vi "Clean exp.vi"(8 "error in (no error)":errorcluster, 11 "Control-Client in":refnum<class "Control-Client.lvclass">) -> (0 "error out":errorcluster, 3 "Control-Client out":refnum<class "Control-Client.lvclass">)   [LabVIEW 2019, in "Control-Client.lvclass"]
uses:
  Control-Client.lvclass
  Control-Client.lvclass/Control-Client.ctl
  Experiments/Experiment.lvclass
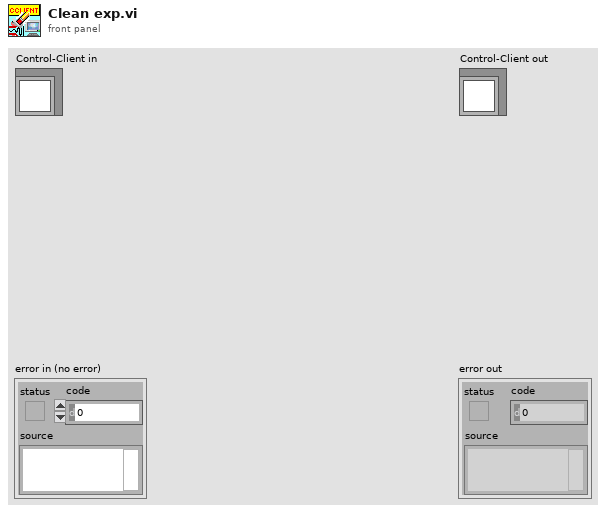
[diagram p1: front panel]
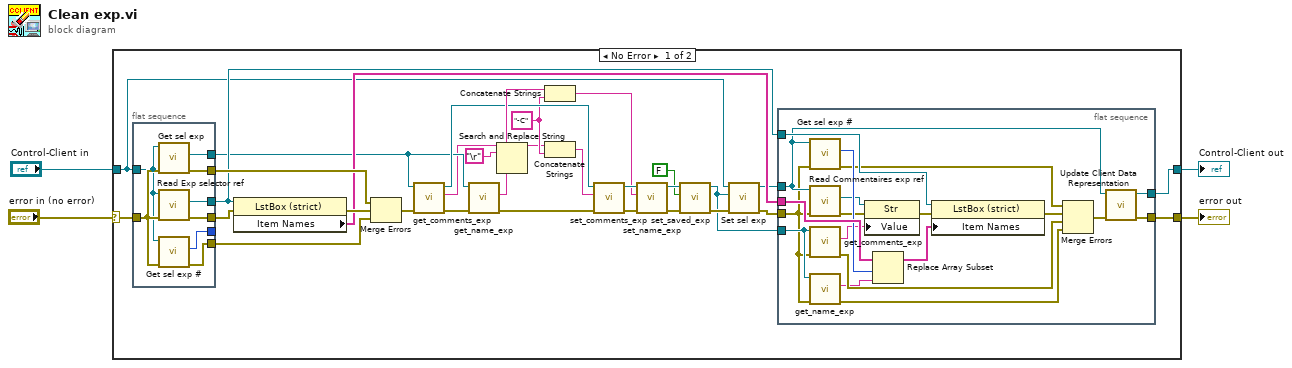
[diagram p0: block diagram]
diagram:
  n1 = case shown="No Error" "error in (no error)" {
    selector: "error in (no error)" -> [w8 w64]
    tunnel: [w9 w64] -> w3
    tunnel: [w10 w63] -> w1
    tunnel: "Control-Client in" -> [w11 w63]
    frame No Error {
      w23 = "-C" ("string")
      n2 = flat-sequence {
        tunnel: [w62] -> w15
        tunnel: [w61] -> w35
        tunnel: [w60] -> w33
        tunnel: w8 -> [w59]
        tunnel: w11 -> [w58]
        tunnel: [w57] -> _
        tunnel: [w56] -> w18
        tunnel: [w55] -> w16
        frame #0 {
          n3 = call "Get sel exp.vi"("error in (no error)"=w59, "Control-Client in"=w58) -> ("error out"=w61:errorcluster, "Sel experiment"=w62:refnum<class "Experiment.lvclass">)  [unwired: 7 in, 1 out]
          n4 = call "Read Exp selector ref.vi"("error in (no error)"=w59, "Control-Client in"=w58) -> ("error out"=w55:errorcluster, "Exp selector ref"=w56:refnum<vi>)  [unwired: 7 in, 1 out]
          n5 = call "Get sel exp #.vi"("error in (no error)"=w59, "Control-Client in"=w58) -> ("error out"=w60:errorcluster, "Exp sel #"=w57:i32)  [unwired: 7 in, 1 out]
        }
      }
      n6 = property on="Property Node" class="LstBox (strict)"(reference=w18, error in=w16) -> (error out=w34:errorcluster, "Item Names"=w19:string[])  [unwired: 1 out]
      n7 = Merge Errors(w35, w34, w33) -> (w14:errorcluster)
      n8 = call "get_comments_exp.vi"("error in (no error)"=w14, "Experiment.lvclass in"=w15) -> ("error out"=w31:errorcluster, "Comments"=w6:string, "Experiment.lvclass out"=w29:refnum<class "Experiment.lvclass">)  [unwired: 7 in]
      n9 = call "get_name_exp.vi"("error in (no error)"=w31, "Experiment.lvclass in"=w15) -> ("error out"=w32:errorcluster, "Exp name"=w30:string)  [unwired: 7 in, 1 out]
      n10 = Search and Replace String(input string=w6, search string="\r") -> (result string=w5:string)  [unwired: 6 in, 3 out]
      n11 = Concatenate Strings(w30, w23) -> (w22:string)
      n12 = Concatenate Strings(w5, w23) -> (w28:string)
      n13 = call "set_comments_exp.vi"("error in (no error)"=w32, "Comments"=w28, "Experiment.lvclass in"=w29) -> ("error out"=w26:errorcluster, "Experiment.lvclass out"=w27:refnum<class "Experiment.lvclass">)  [unwired: 7 in]
      n14 = call "set_name_exp.vi"("error in (no error)"=w26, "Exp name"=w22, "Experiment.lvclass in"=w27) -> ("error out"=w24:errorcluster, "Experiment.lvclass out"=w25:refnum<class "Experiment.lvclass">)  [unwired: 7 in]
      n15 = call "set_saved_exp.vi"("error in (no error)"=w24, "Saved"=FALSE, "Experiment.lvclass in"=w25) -> ("error out"=w20:errorcluster, "Experiment.lvclass out"=w17:refnum<class "Experiment.lvclass">)  [unwired: 7 in]
      n16 = call "Set sel exp.vi"("error in (no error)"=w20, "Experiment"=w17, "Control-Client in"=w11) -> ("error out"=w12:errorcluster, "Control-Client out"=w13:refnum<class "Control-Client.lvclass">)  [unwired: 7 in]
      n17 = flat-sequence {
        tunnel: w19 -> [w54]
        tunnel: w18 -> [w53]
        tunnel: w17 -> [w52]
        tunnel: w13 -> [w51]
        tunnel: w12 -> [w50]
        tunnel: [w49] -> w10
        tunnel: [w48] -> w9
        frame #0 {
          n18 = call "Get sel exp #.vi"("error in (no error)"=w50, "Control-Client in"=w51) -> ("error out"=w39:errorcluster, "Exp sel #"=w46:i32)  [unwired: 7 in, 1 out]
          n19 = call "Read Commentaires exp ref.vi"("error in (no error)"=w50, "Control-Client in"=w51) -> ("error out"=w43:errorcluster, "Commentaires exp ref"=w45:refnum<vi>)  [unwired: 7 in, 1 out]
          n20 = call "get_comments_exp.vi"("error in (no error)"=w50, "Experiment.lvclass in"=w52) -> ("error out"=w41:errorcluster, "Comments"=w44:string)  [unwired: 7 in, 1 out]
          n21 = call "get_name_exp.vi"("error in (no error)"=w50, "Experiment.lvclass in"=w52) -> ("error out"=w36:errorcluster, "Exp name"=w38:string)  [unwired: 7 in, 1 out]
          n22 = property on="Property Node" class="Str"(reference=w45, error in=w43, "Value"=w44) -> (error out=w42:errorcluster)  [unwired: 1 out]
          n23 = Replace Array Subset(array=w54, new element=w38, index=w46) -> (w47:string[])
          n24 = property on="Property Node" class="LstBox (strict)"(reference=w53, error in=w42, "Item Names"=w47) -> (error out=w40:errorcluster)  [unwired: 1 out]
          n25 = Merge Errors(w39, w40, w41, w36) -> (w37:errorcluster)
          n26 = call "Update Client Data Representation.vi"("error in (no error)"=w37, "Control-Client in"=w51) -> ("error out"=w48:errorcluster, "Control-Client out"=w49:refnum<class "Control-Client.lvclass">)  [unwired: 8 in]
        }
      }
    }
    frame Error {
    }
  }
  "error out" <- w3
  "Control-Client out" <- w1
